vi "RotateArray.vi"(6 "Vel grid Ideal":cdb[][](array[numeric]), 7 "Pad Pts":i32=1, 8 "Peak V in":dbl[][](graph), 10 "Header In":T1 {"Compression Parameters"."% taper" min=50 max=1000 format="%.2f"; "Compression Parameters"."F2 (MHz)" format="%.3f"; "Compression Parameters"."F1 (MHz)" format="%.3f"; "Scan Settings"."prf (kHz)" format="%.2f"; "Therapy Parameters"."Therapy amplitude (mV)" min=50 max=1000 format="%.2f"; "Therapy Parameters"."Time on (s)" format="%.3f"; "Therapy Parameters"."Theraputic Freq (MHz)" format="%.3f"; "Patient Info"."Race" items=["Am Ind or Alaska", "Asian", "Hawaiian, Pac Isl", "Black or Afr Amer", "White", "more than one race", "unknown"]; "Patient Info"."Ethnicty 2" items=["Hispanic", "Non-Hispanic", "unknown"]; "Patient Info"."LOS" items=["1", "2", "3", "4", "5"]; "Patient Info"."PSA" format="%.1f"; "Scan Info"."delay" format="%.2f"; "Scan Info"."pivot distance" format="%.2f"; "Scan Info"."sector scan angle" format="%.2f"; "Tranducer Info"."bandwidth" format="%.2f"; "Tranducer Info"."center freq" format="%.2f"; "Tranducer Info"."start freq" format="%.2f"}, 11 "Angle":dbl) -> (2 "Dop Spec":sgl[](graph), 3 "Peak V out":dbl[][](graph))   [LabVIEW 2022 SP3]
uses:
  ViewData/-ReadEye/Header.ctl
  <vilib>/Analysis/1siggen.llb/Ramp Pattern by Samples.vi
  <vilib>/Analysis/baseanly.llb/Mean (DBL).vi
  <vilib>/gmath/interp.llb/Interpolate 2D (2d X,Y).vi
  <vilib>/gmath/interp.llb/Create Mesh Grid (2D) (x,y arrays).vi
  <vilib>/gmath/interp.llb/Interpolate 2D (1d X,Y).vi
  <vilib>/gmath/NI_Gmath.lvlib
  <vilib>/Analysis/NI_AALBase.lvlib
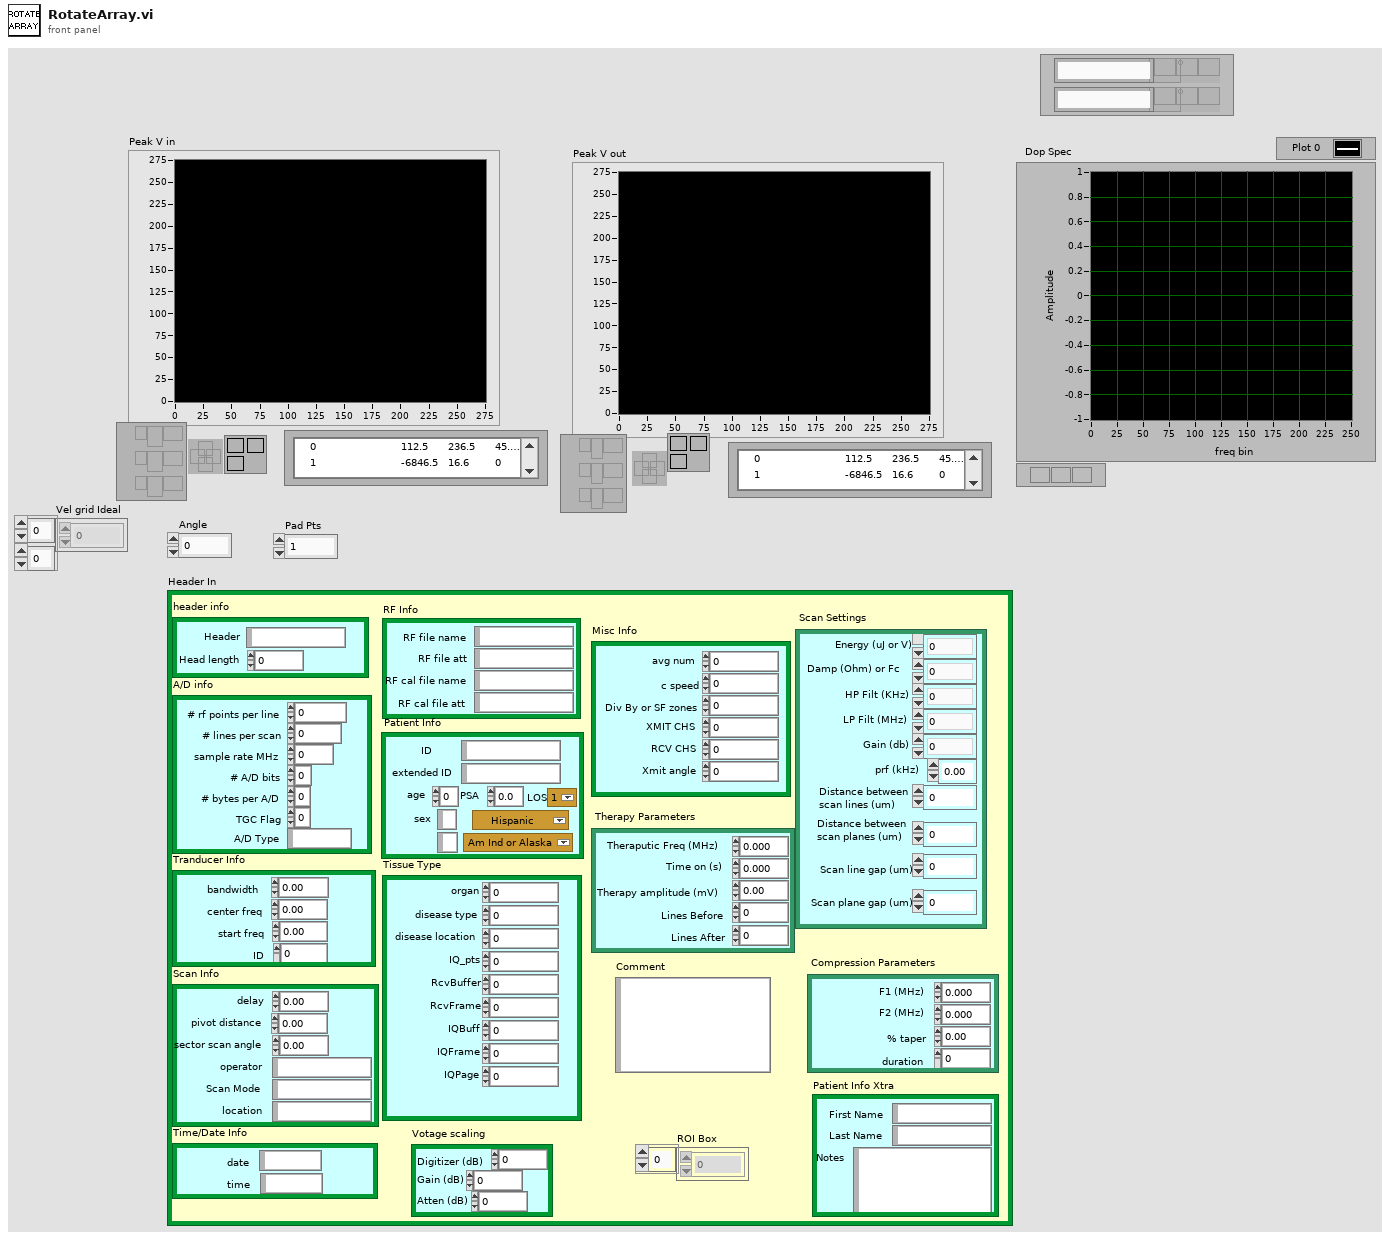
[diagram p1: front panel]
types:
  T1 = typedef "Header.ctl" = cluster{"header info":cluster{"Header":string, "Head length":i16}, "A/D info":cluster{"# rf points per line":u16, "# lines per scan":u16, "sample rate MHz":u16, "# A/D bits":i16, "# bytes per A/D":u16, "TGC Flag":u16, "A/D Type":string}, "Tranducer Info":cluster{"bandwidth":sgl, "center freq":sgl, "start freq":sgl, "ID":i32}, "Scan Info":cluster{"delay":sgl, "pivot distance":sgl, "sector scan angle":sgl, "operator":string, "Scan Mode":string, "location":string}, "Time/Date Info":cluster{"date":string, "time":string}, "RF Info":cluster{"RF file name":string, "RF file att":string, "RF cal file name":string, "RF cal file att":string}, "Patient Info":cluster{"ID":string, "extended ID":string, "age":u16, "sex":string, "previously\nscanned":string, "PSA":sgl, "LOS":u8, "Ethnicty 2":u8, "Race":u8}, "Tissue Type":cluster{"organ":i16, "disease type":i16, "disease location":i16, "IQ_pts":u16, "RcvBuffer":u8, "RcvFrame":u16, "IQBuff":u8, "IQFrame":u16, "IQPage":u8}, "Votage scaling":cluster{"Digitizer (dB)":sgl, "Gain (dB)":sgl, "Atten (dB)":sgl}, "Comment":string, "Misc Info":cluster{"avg num":u16, "c speed":i16, "Div By or SF zones":i16, "XMIT CHS":u8, "RCV CHS":u8, "Xmit angle":sgl}, "Therapy Parameters":cluster{"Theraputic Freq (MHz)":sgl, "Time on (s)":sgl, "Therapy amplitude (mV)":sgl, "Lines Before":u16, "Lines After":u16}, "Scan Settings":cluster{"Energy (uJ or V)":u8, "Damp (Ohm) or Fc":u8, "HP Filt (KHz)":u8, "LP Filt (MHz)":u8, "Gain (db)":u8, "prf (kHz)":sgl, "Distance between\nscan lines (um)":u16, "Distance between\nscan planes (um)":u16, "Scan line gap (um)":sgl, "Scan plane gap (um)":sgl}, "Compression Parameters":cluster{"F1 (MHz)":sgl, "F2 (MHz)":sgl, "% taper":sgl, "duration":sgl}, "Patient Info Xtra":cluster{"First Name":string, "Last Name":string, "Notes":string}, "ROI Box":u16[]}
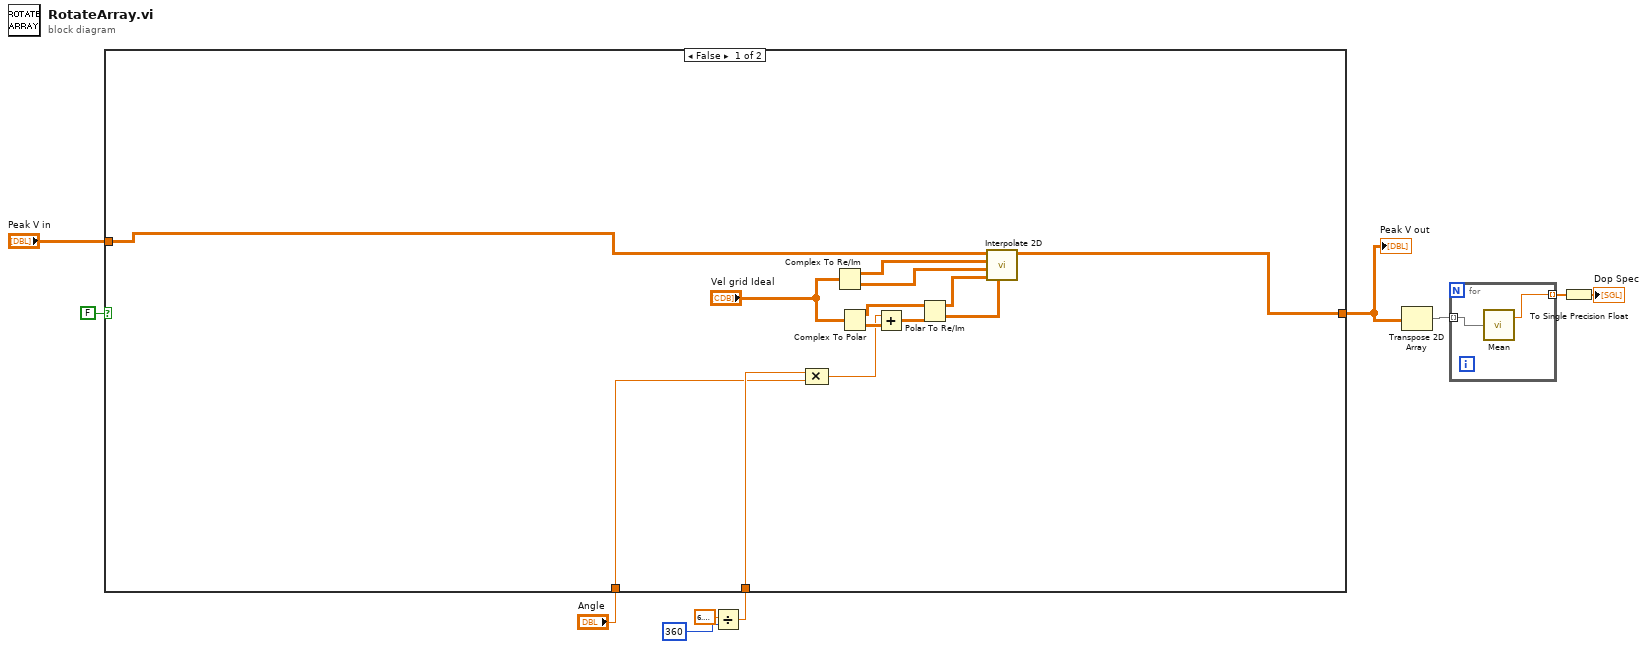
[diagram p0: block diagram]
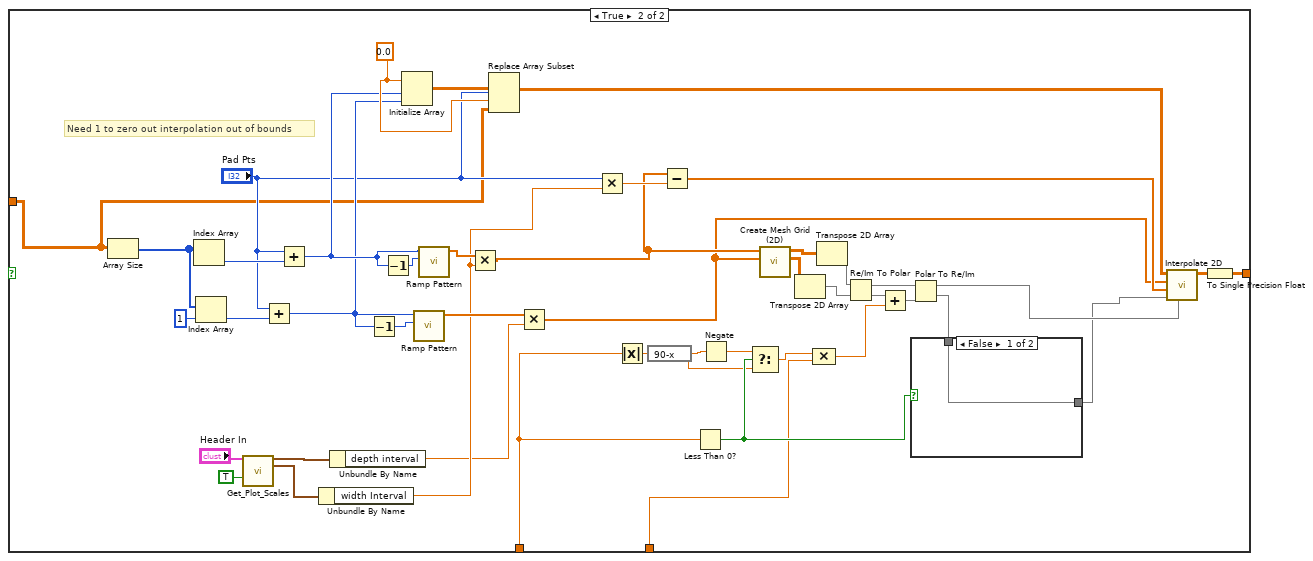
[diagram p2: hidden frame]
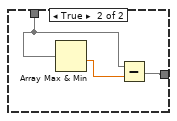
[diagram p3: hidden frame]
diagram:
  n1 = Divide(x=6.283185307179586, y=360) -> (x/y=w3:dbl)
  n2 = case shown="False" FALSE {
    tunnel: "Peak V in" -> [w11 w31]
    tunnel: [w16 w30] -> w6
    tunnel: "Angle" -> [w13 w25]
    tunnel: w3 -> [w15 w24]
    frame False {
      n3 = Compound Arithmetic op=MULTIPLY(w15, w13) -> (w14:dbl)
      n4 = Complex To Re/Im(x + iy="Vel grid Ideal") -> (x=w17:dbl[][], y=w18:dbl[][])
      n5 = Complex To Polar(r * e^(i*theta)="Vel grid Ideal") -> (r=w21:dbl[][], theta=w19:dbl[][])
      n6 = Add(x=w14, y=w19) -> (x+y=w20:dbl[][])
      n7 = Polar To Re/Im(2:w20, 3:w21) -> (0:w23:dbl[][], 1:w22:dbl[][])
      n8 = call-poly <vilib>:"Interpolate 2D.vi"("yi"=w23, "xi"=w22, "Y"=w18, "X"=w17, "Z"=w11) -> ("zi"=w16:dbl[][])  [unwired: 3 in, 3 out]
    }
    frame True {
      w50 = 0.0 ("index")
      # "Need 1 to zero out interpolation out of bounds"
      n9 = Array Size(array=w31) -> (size(s)=w67:i32[])
      n10 = Index Array(array=w67) -> (element=w52:i32)  [unwired: 1 in]
      n11 = Index Array(array=w67, index=1) -> (element=w45:i32)
      n12 = call "Get_Plot_Scales.vi"("Header In"="Header In", "Axis scaling"=TRUE) -> ("Depth Scale"=w26:cluster{"start depth":dbl, "depth interval":dbl}, "Width Scale"=w27:cluster{"Start":dbl, "width Interval":dbl})  [unwired: 12 in]
      n13 = Add(x="Pad Pts", y=w45) -> (x+y=w43:i32)
      n14 = Add(x="Pad Pts", y=w52) -> (x+y=w46:i32)
      n15 = Unbundle By Name(w27) -> ("width Interval"=w49:dbl)
      n16 = Unbundle By Name(w26) -> ("depth interval"=w47:dbl)
      n17 = Decrement(x=w43) -> (x-1=w54:i32)
      n18 = Decrement(x=w46) -> (x-1=w55:i32)
      n19 = Initialize Array(w50, w46, w43) -> (w51:dbl[][])
      n20 = call-poly <vilib>:"Ramp Pattern.vi"("end"=w54, "samples"=w43) -> ("Ramp Pattern"=w57:dbl[])  [unwired: 8 in, 1 out]
      n21 = call-poly <vilib>:"Ramp Pattern.vi"("end"=w55, "samples"=w46) -> ("Ramp Pattern"=w58:dbl[])  [unwired: 8 in, 1 out]
      n22 = Multiply(x=w58, y=w49) -> (x*y=w35:dbl[])
      n23 = Replace Array Subset(array=w51, new element=w31, index (row)="Pad Pts", index (col)=w50) -> (w44:dbl[][])
      n24 = Multiply(x=w57, y=w47) -> (x*y=w34:dbl[])
      n25 = Multiply(x="Pad Pts", y=w49) -> (x*y=w48:dbl)
      n26 = Absolute Value(x=w25) -> (abs(x)=w40:dbl)
      n27 = expression code="90-x"(w40) -> (w38:dbl)
      n28 = Subtract(x=w35, y=w48) -> (x-y=w42:dbl[])
      n29 = Less Than 0?(x=w25) -> (x < 0?=w39:bool)
      n30 = Negate(x=w38) -> (-x=w37:dbl)
      n31 = Select(t=w37, s=w39, f=w38) -> (s? t:f=w32:dbl)
      n32 = call-poly <vilib>:"Create Mesh Grid (2D).vi"("y domain"=w34, "x domain"=w35) -> ("Y"=w63:dbl[][], "X"=w62:dbl[][])  [unwired: 7 in, 1 out]
      n33 = Transpose 2D Array(2D array=w63) -> (transposed array=w60:dbl[][])
      n34 = Compound Arithmetic op=MULTIPLY(w32, w24) -> (w56:dbl)
      n35 = Transpose 2D Array(2D array=w62) -> (transposed array=w61:dbl[][])
      n36 = Re/Im To Polar(2:w60, 3:w61) -> (0:w66:dbl[][], 1:w64:dbl[][])
      n37 = Add(x=w66, y=w56) -> (x+y=w65:dbl[][])
      n38 = Polar To Re/Im(2:w65, 3:w64) -> (0:w36:dbl[][], 1:w53:dbl[][])
      n39 = case shown="False" w39 {
        tunnel: w36 -> [w69 w71]
        tunnel: [w69 w70] -> w33
        frame False {
        }
        frame True {
          n40 = Array Max & Min(array=w71) -> (min value=w72:dbl)  [unwired: 3 out]
          n41 = Subtract(x=w71, y=w72) -> (x-y=w70:dbl[][])
        }
      }
      n42 = call-poly <vilib>:"Interpolate 2D.vi"("yi"=w53, "xi"=w33, "Y"=w42, "X"=w34, "Z"=w44) -> ("zi"=w59:dbl[][])  [unwired: 3 in, 3 out]
      n43 = To Single Precision Float(number=w59) -> (single precision float=w30:sgl[][])
    }
  }
  "Peak V out" <- w6
  n44 = Transpose 2D Array(2D array=w6) -> (transposed array=w7:dbl[][])
  n45 = for {
    tunnel: w7 -> [w74] mode=indexing
    tunnel: [w73] -> w8 mode=indexing
    n46 = call-poly <vilib>:"Mean.vi"("X"=w74) -> ("mean"=w73:dbl)  [unwired: 1 out]
  }
  n47 = To Single Precision Float(number=w8) -> (single precision float=→"Dop Spec":sgl[])
